vi "Initialize.vi"(8 "error in (no error)":errorcluster, 11 "GRMActor in":refnum<class "FlatField.lvclass">) -> (0 "error out":errorcluster, 3 "GRMActor out":refnum<class "FlatField.lvclass">)   [LabVIEW 2020, in "FlatField.lvlib" / "FlatField.lvclass"]
uses:
  FlatField.lvclass
  FlatField Status.ctl
  FlatField.lvclass/FlatField.ctl
  Model/Hardware Abstraction Layer/Component/GenericActor/GenericActor/GenericActor.lvclass
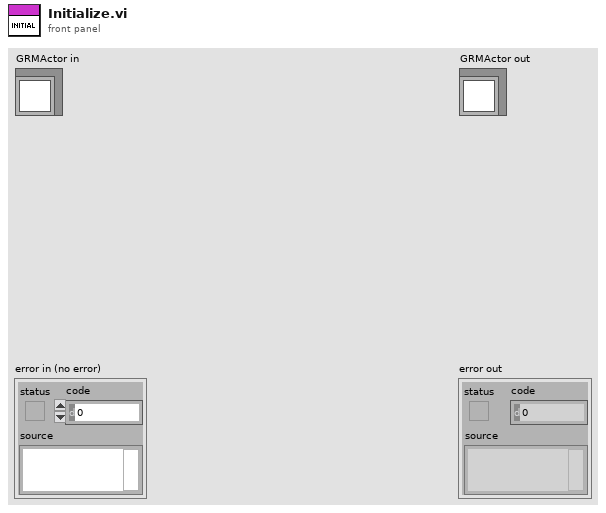
[diagram p1: front panel]
types:
  T1 = typedef "Image Type" = u32
  T2 = typedef "FlatField.lvlib/FlatField.lvclass/FlatField Status.ctl" = i32
  T3 = typedef "IMAQ Image.ctl" = refnum<image>
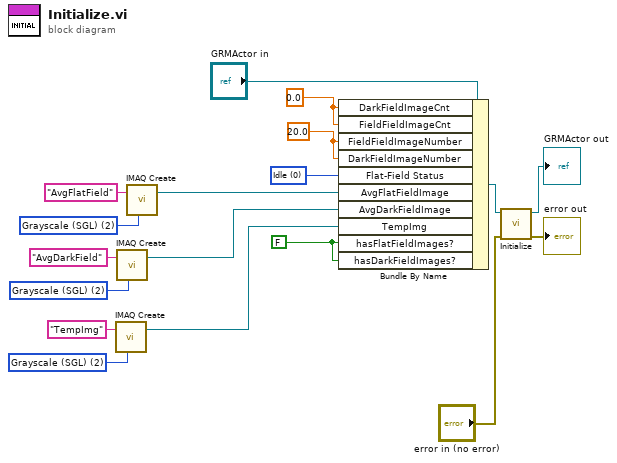
[diagram p0: block diagram]
diagram:
  w1 = FALSE ("hasFlatFieldImages?")
  w3 = T1 2 items=["Grayscale (U8)", "Grayscale (I16)", "Grayscale (SGL)", "Complex (CSG)", "RGB (U32)", "HSL (U32)", "RGB (U64)", "Grayscale (U16)"] ("Image Type")
  w7 = T1 2 items=["Grayscale (U8)", "Grayscale (I16)", "Grayscale (SGL)", "Complex (CSG)", "RGB (U32)", "HSL (U32)", "RGB (U64)", "Grayscale (U16)"] ("Image Type")
  w8 = T1 2 items=["Grayscale (U8)", "Grayscale (I16)", "Grayscale (SGL)", "Complex (CSG)", "RGB (U32)", "HSL (U32)", "RGB (U64)", "Grayscale (U16)"] ("Image Type")
  w11 = 0.0 ("DarkFieldImageCnt")
  w12 = 20.0 ("FieldFieldImageNumber")
  w13 = T2 0 items=["Idle", "Taking DarkField Images", "Taking FlatField Image", "Doing FlatField", ""] ("Flat-Field Status")
  n1 = call "IMAQ Create"("Image Name"="TempImg", "Image Type"=w3) -> ("New Image"=w2:T3)  [unwired: 3 in, 1 out]
  n2 = call "IMAQ Create"("Image Name"="AvgDarkField", "Image Type"=w7) -> ("New Image"=w5:T3)  [unwired: 3 in, 1 out]
  n3 = call "IMAQ Create"("Image Name"="AvgFlatField", "Image Type"=w8) -> ("New Image"=w10:T3)  [unwired: 3 in, 1 out]
  n4 = Bundle By Name(cluster="GRMActor in", "DarkFieldImageCnt"=w11, "FieldFieldImageCnt"=w11, "FieldFieldImageNumber"=w12, "DarkFieldImageNumber"=w12, "Flat-Field Status"=w13, "AvgFlatFieldImage"=w10, "AvgDarkFieldImage"=w5, "TempImg"=w2, "hasFlatFieldImages?"=w1, "hasDarkFieldImages?"=w1) -> (w14:refnum<class "FlatField.lvclass">)
  n5 = call-parent "Initialize.vi"("error in (no error)"="error in (no error)", "GRMActor in"=w14) -> ("error out"=→"error out":errorcluster, "GRMActor out"=→"GRMActor out":refnum<class "FlatField.lvclass">)  [unwired: 8 in]
